vi "Shift_Value_CH1_calibration_Rev02x.vi"(0 "Saved Val IN2":dbl, 1 "Enable memory wright":bool, 3 "INPUT2 R range in":dbl, 4 "USB Interface Name":refnum<visa-resource-name>="COM3", 5 "Input buffer size":u32=16384, 6 "Cal Voltage IN2":dbl, 7 "error in (no error)":errorcluster, 13 "WRITE":bool, 27 "Sign Value":dbl) -> (8 "MB address":string, 9 "MB value":u8 format="%x", 11 "Cal to Saved IN2":dbl, 12 "UB address":string, 14 "HB address":string, 15 "error out":errorcluster, 16 "LB address":string, 17 "UB value":u8 format="%x", 18 "Reply 1":string, 19 "Reply 4":string, 20 "CH1 shift value uV":dbl, 21 "CH1shift val HEX uV":u32 format="%x", 22 "Reply 2":string, 23 "Sign Addrss":string, 24 "HB value":u8 format="%x", 25 "LB value":u8 format="%x", 26 "Reply 3":string)   [LabVIEW 2012]
panel:
  out "LB value":string
  out "HB value":string
  out "UB value":string
  out "MB value":string
  # "1. Computes address based on the input range \"Range IN\"\n2. Take absolute values of positive and negative voltage reads in uV compares them and subtracts smaller value from the larger one. The result is devided by 2.\nIf VAL1>VAL2: ( |VAL1| - |VAL2| )/ 2"
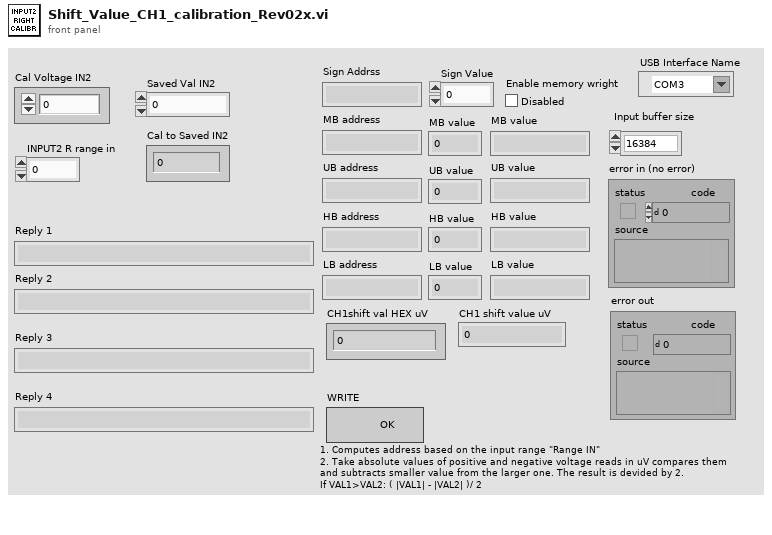
[diagram p1: front panel]
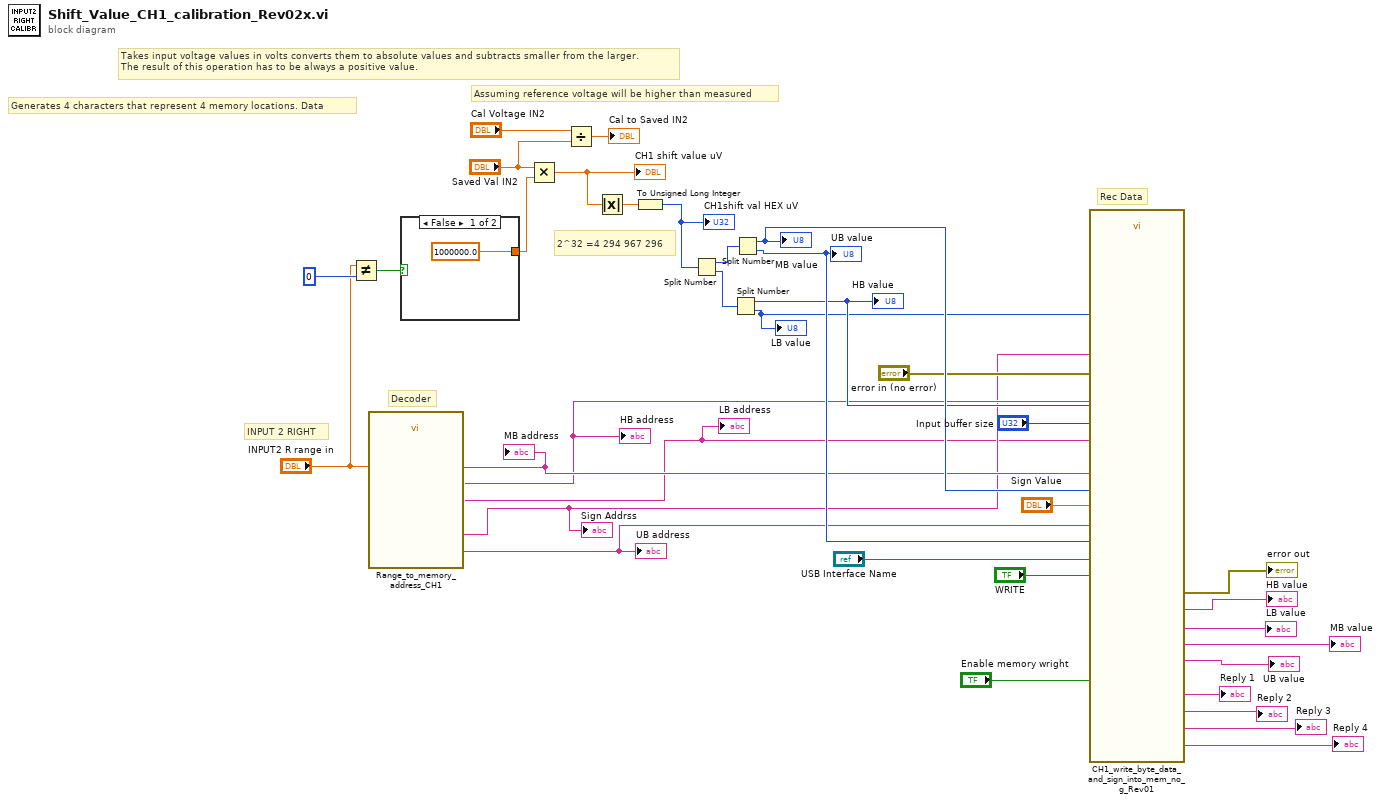
[diagram p0: block diagram]
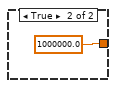
[diagram p2: hidden frame]
diagram:
  # "Rec Data"
  # "Decoder"
  # "Assuming reference voltage will be higher than measured"
  # "INPUT 2 RIGHT"
  # "2^32 =4 294 967 296"
  # "Generates 4 characters that represent 4 memory locations. Data"
  # "Takes input voltage values in volts converts them to absolute values and subtracts smaller from the larger.\nThe result of this operation has to be always a positive value."
  n1 = Not Equal?(x="INPUT2 R range in", y=0) -> (x != y?=w7:bool)
  n2 = call "Range_to_memory_address_CH1.vi"("INPUT2 CH1 Range IN"="INPUT2 R range in") -> ("LB address"=w11:string, "HB address"=w18:string, "UB address"=w19:string, "MB address"=w20:string, "Sign Addrss"=w17:string)  [unwired: 6 in]
  "MB address" <- w20
  "UB address" <- w19
  "HB address" <- w18
  "LB address" <- w11
  "Sign Addrss" <- w17
  n3 = case shown="False" w7 {
    tunnel: [1000000.0 1000000.0] -> w5
    frame False {
    }
    frame True {
    }
  }
  n4 = Multiply(x="Saved Val IN2", y=w5) -> (x*y=w14:dbl)
  "CH1 shift value uV" <- w14
  n5 = Divide(x="Cal Voltage IN2", y="Saved Val IN2") -> (x/y=→"Cal to Saved IN2":dbl)
  n6 = Absolute Value(x=w14) -> (abs(x)=w15:dbl)
  n7 = To Unsigned Long Integer(number=w15) -> (unsigned 32bit integer=w16:u32)
  "CH1shift val HEX uV" <- w16
  n8 = Split Number(x=w16) -> (hi(x)=w36:u16, lo(x)=w35:u16)
  n9 = Split Number(x=w35) -> (hi(x)=w29:u8, lo(x)=w28:u8)
  "HB value" <- w29
  "LB value" <- w28
  n10 = Split Number(x=w36) -> (hi(x)=w34:u8, lo(x)=w30:u8)
  "MB value" <- w34
  "UB value" <- w30
  n11 = call "CH1_write_byte_data_and_sign_into_mem_no_g_Rev01.vi"("MB data"=w34, "UB data"=w30, "Address of the sign"=w17, "USB Interface Name"="USB Interface Name", "HB data"=w29, "LB data"=w28, "MB address"=w20, "HB address"=w18, "LB address"=w11, "Sign Value"="Sign Value", "WRITE DATA"="WRITE", "Input buffer size"="Input buffer size", "UB address"=w19, "error in (no error)"="error in (no error)", "Enable memory wright"="Enable memory wright") -> ("Reply 1"=→"Reply 1":string, "Reply 4"=→"Reply 4":string, "MB data string"=→"MB value":string, "UB data string"=→"UB value":string, "Reply 2"=→"Reply 2":string, "error out"=→"error out":errorcluster, "HB data string"=→"HB value":string, "Reply 3"=→"Reply 3":string, "LB data string"=→"LB value":string)  [unwired: 4 in]
